vi "Boolean Strings.vi"(8 "Enum":enum16{"List", "Add", "Remove"}(ring), 9 "Customer False Boolean Strings":string[](array[string]), 10 "Customer True Boolean Strings":string[](array[string])) -> (0 "Numeric":i32, 1 "False Boolean Strings":string[](array[string]), 2 "True Boolean Strings":string[](array[string]), 3 "Array":string[](array[string]))   [LabVIEW 2017, in "API String Arguments Support.lvlib"]
uses:
  API String Arguments Support.lvlib
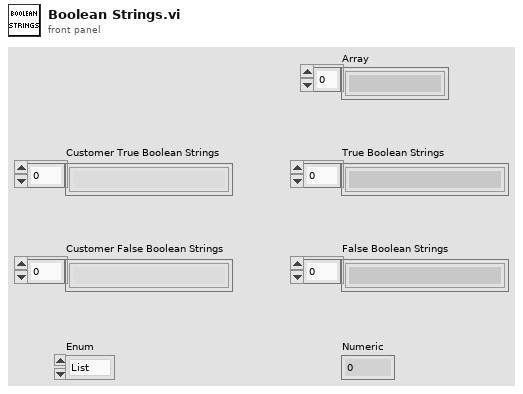
[diagram p1: front panel]
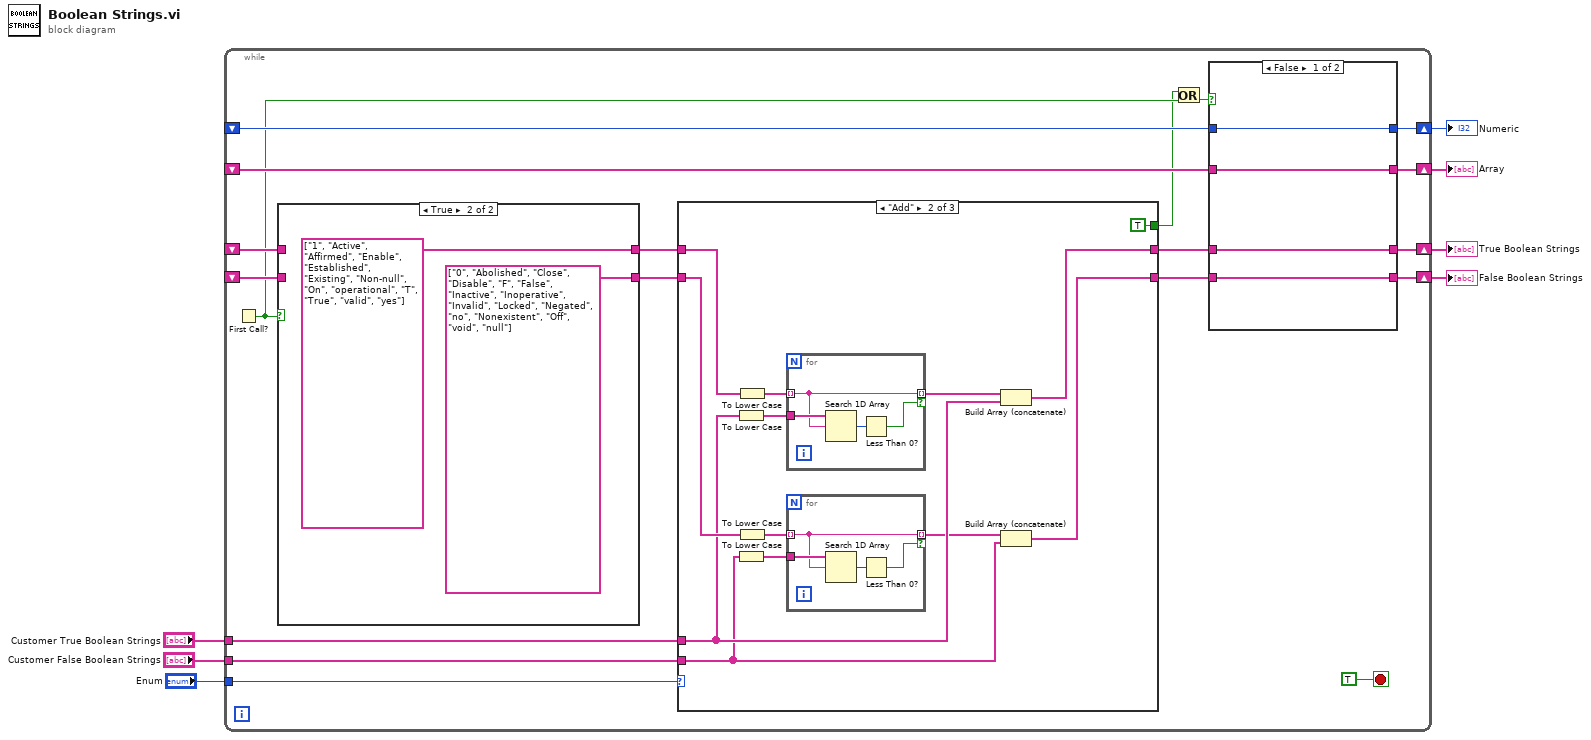
[diagram p0: block diagram]
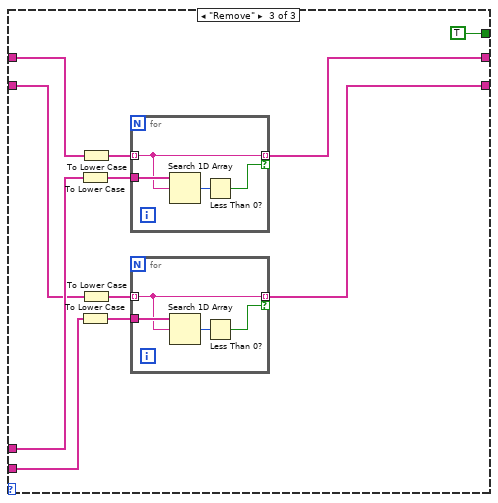
[diagram p4: hidden frame]
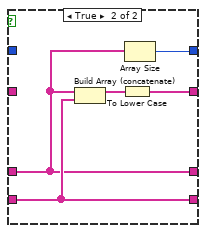
[diagram p5: hidden frame]
diagram:
  n1 = while {
    tunnel: "Enum" -> [w25]
    shift-right: [w17] -> w7
    shift-left: _ -> [w16]
    shift-right: [w15] -> w2
    shift-left: _ -> [w22]
    shift-right: [w13] -> w1
    shift-left: _ -> [w21]
    shift-right: [w18] -> w6
    shift-left: _ -> [w11]
    tunnel: "Customer True Boolean Strings" -> [w20]
    tunnel: "Customer False Boolean Strings" -> [w19]
    stop <- TRUE stop-if-true
    n2 = First Call?() -> (First Call?: T/F=w10:bool)
    n3 = case shown="True" w10 {
      tunnel: [w28 string[] ["1", "Active", "Affirmed", "Enable", "Established", "Existing", "Non-null", "On", "operational", "T", "True", "valid", "yes"]] -> w24
      tunnel: [w27 string[] ["0", "Abolished", "Close", "Disable", "F", "False", "Inactive", "Inoperative", "Invalid", "Locked", "Negated", "no", "Nonexistent", "Off", "void", "null"]] -> w23
      tunnel: w22 -> [w28 _]
      tunnel: w21 -> [w27 _]
      frame False {
      }
      frame True {
      }
    }
    n4 = case shown="\"Add\"" w25 {
      tunnel: w24 -> [w32 w35 w63]
      tunnel: w23 -> [w31 w40 w57]
      tunnel: [w32 w34 w55] -> w14
      tunnel: [w31 w33 w54] -> w12
      tunnel: w20 -> [_ w38 w62]
      tunnel: w19 -> [_ w36 w56]
      tunnel: [_ TRUE ("x") TRUE ("x")] -> w8
      frame "List", Default {
      }
      frame "Add" {
        n5 = To Lower Case(string=w38) -> (all lower case string=w43:string[])
        n6 = To Lower Case(string=w36) -> (all lower case string=w42:string[])
        n7 = To Lower Case(string=w35) -> (all lower case string=w44:string[])
        n8 = To Lower Case(string=w40) -> (all lower case string=w41:string[])
        n9 = for {
          tunnel: w44 -> [w52] mode=indexing
          tunnel: w43 -> [w53]
          tunnel: [w52] -> w39 mode=indexing if=w50
          n10 = Search 1D Array(1D array=w53, element=w52) -> (index of element=w51:i32)  [unwired: 1 in]
          n11 = Less Than 0?(x=w51) -> (x < 0?=w50:bool)
        }
        n12 = for {
          tunnel: w41 -> [w48] mode=indexing
          tunnel: w42 -> [w49]
          tunnel: [w48] -> w37 mode=indexing if=w46
          n13 = Search 1D Array(1D array=w49, element=w48) -> (index of element=w47:i32)  [unwired: 1 in]
          n14 = Less Than 0?(x=w47) -> (x < 0?=w46:bool)
        }
        n15 = Build Array (concatenate)(w39, w38) -> (w34:string[])
        n16 = Build Array (concatenate)(w37, w36) -> (w33:string[])
      }
      frame "Remove" {
        n17 = To Lower Case(string=w62) -> (all lower case string=w60:string[])
        n18 = To Lower Case(string=w56) -> (all lower case string=w59:string[])
        n19 = To Lower Case(string=w63) -> (all lower case string=w61:string[])
        n20 = To Lower Case(string=w57) -> (all lower case string=w58:string[])
        n21 = for {
          tunnel: w61 -> [w71] mode=indexing
          tunnel: w60 -> [w72]
          tunnel: [w71] -> w55 mode=indexing if=w69
          n22 = Search 1D Array(1D array=w72, element=w71) -> (index of element=w70:i32)  [unwired: 1 in]
          n23 = Less Than 0?(x=w70) -> (x < 0?=w69:bool)
        }
        n24 = for {
          tunnel: w58 -> [w67] mode=indexing
          tunnel: w59 -> [w68]
          tunnel: [w67] -> w54 mode=indexing if=w65
          n25 = Search 1D Array(1D array=w68, element=w67) -> (index of element=w66:i32)  [unwired: 1 in]
          n26 = Less Than 0?(x=w66) -> (x < 0?=w65:bool)
        }
      }
    }
    n27 = Or(x=w8, y=w10) -> (x .or. y?=w9:bool)
    n28 = case shown="False" w9 {
      tunnel: [w76 w80] -> w18
      tunnel: [w75 w79] -> w17
      tunnel: w16 -> [w75 _]
      tunnel: [w74 w77] -> w15
      tunnel: w14 -> [w74 w77]
      tunnel: [w73 w78] -> w13
      tunnel: w12 -> [w73 w78]
      tunnel: w11 -> [w76 _]
      frame False {
      }
      frame True {
        n29 = Build Array (concatenate)(w77, w78) -> (w81:string[])
        n30 = To Lower Case(string=w81) -> (all lower case string=w79:string[])
        n31 = Array Size(array=w77) -> (size(s)=w80:i32)
      }
    }
  }
  "Numeric" <- w6
  "Array" <- w7
  "True Boolean Strings" <- w2
  "False Boolean Strings" <- w1
